vi "7p1_HW_Task1C_doanbs.vi"(9 "x, Original Value":dbl, 10 "Output in Degrees or Radians?":string, 11 "Inverse Trig Function":string) -> (2 "th, Theta":dbl, 3 "Units":string)   [LabVIEW 2016]
uses:
  <vilib>/express/express arith-compare/Formula/XNode/ExpressFormulaBlockNode.xnode
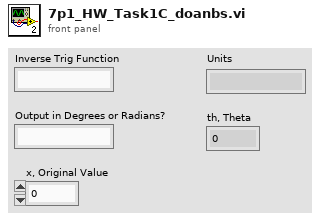
[diagram p1: front panel]
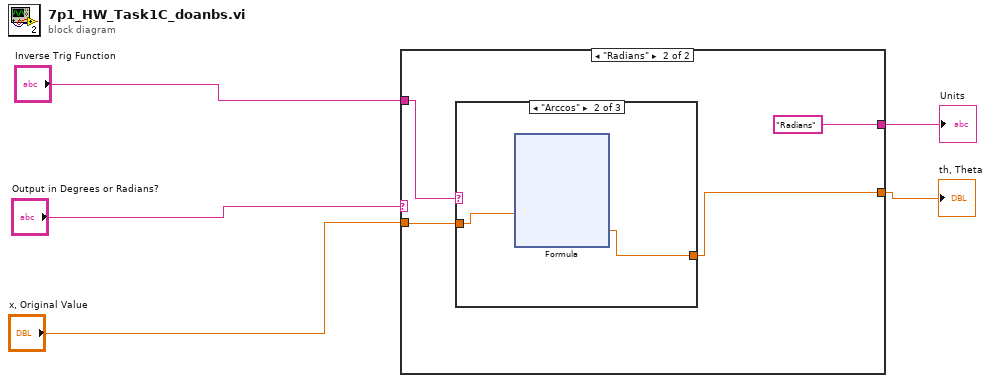
[diagram p0: block diagram]
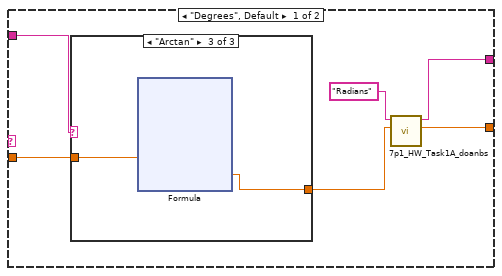
[diagram p2: hidden frame]
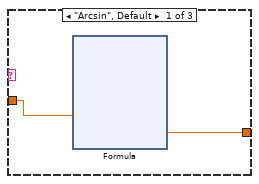
[diagram p3: hidden frame]
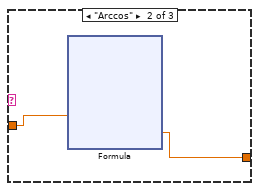
[diagram p4: hidden frame]
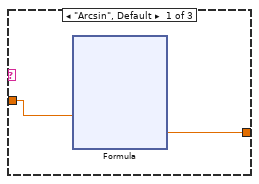
[diagram p5: hidden frame]
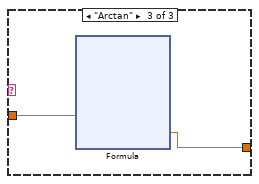
[diagram p6: hidden frame]
diagram:
  n1 = case shown="\"Radians\"" "Output in Degrees or Radians?" {
    tunnel: "Inverse Trig Function" -> [w11 w43]
    tunnel: "x, Original Value" -> [w10 w44]
    tunnel: [w8 w42] -> w4
    tunnel: [w7 "Radians"] -> w5
    frame "Degrees", Default {
      n2 = case shown="\"Arctan\"" w11 {
        tunnel: w10 -> [w13 w23 w33]
        tunnel: [w12 w22 w32] -> w9
        frame "Arcsin", Default {
          n3 = xnode "Formula"("x"=w13) -> ("Result"=w12:dbl)  [unwired: 1 in, 1 out]
        }
        frame "Arccos" {
          n4 = xnode "Formula"("x"=w23) -> ("Result"=w22:dbl)  [unwired: 1 in, 1 out]
        }
        frame "Arctan" {
          n5 = xnode "Formula"("x"=w33) -> ("Result"=w32:dbl)  [unwired: 1 in, 1 out]
        }
      }
      n6 = call "7p1_HW_Task1A_doanbs.vi"("th, Theta in"=w9, "Units in"="Radians") -> ("th, Theta out"=w8:dbl, "Units out"=w7:string)  [unwired: 8 in]
    }
    frame "Radians" {
      n7 = case shown="\"Arccos\"" w43 {
        tunnel: w44 -> [w47 w57 w67]
        tunnel: [w46 w56 w66] -> w42
        frame "Arcsin", Default {
          n8 = xnode "Formula"("x"=w47) -> ("Result"=w46:dbl)  [unwired: 1 in, 1 out]
        }
        frame "Arccos" {
          n9 = xnode "Formula"("x"=w57) -> ("Result"=w56:dbl)  [unwired: 1 in, 1 out]
        }
        frame "Arctan" {
          n10 = xnode "Formula"("x"=w67) -> ("Result"=w66:dbl)  [unwired: 1 in, 1 out]
        }
      }
    }
  }
  "Units" <- w5
  "th, Theta" <- w4
